vi "Drive Controller.vi"(8 "error in":errorcluster) -> ()   [LabVIEW 2018]
doc: "This VI executes continuously carrying out the current operation and responding to updates or new operation requests. It will often contain the timing or control code that is difficult to place directly in TeleOp. This VI generally opens all sensors and motors and isolates the rest of the robot code from knowing implementation details of how the operations are carried out."
uses:
  Drive Operations.ctl
  Drive Setpoints.ctl
  <vilib>/Rock Robotics/WPI/MotorControl/WPI_MotorControlOpen SPARK.vi
  <vilib>/Rock Robotics/SystemInterfaces/DIO/FPGA_DIOPWMChannel.ctl
  <vilib>/Rock Robotics/WPI/Framework/Completion Status.ctl
panel:
  in  "Interactive Values":T1
  in  "Buttons":cluster{"Execute Cmd":bool, "Abort Cmd":bool}
  out "Command Timing":cluster{"Start Time (ms)":u32, "Iterations":i32}
  out "Status":T3
  out "Current\nCmd":string
  # "Tip: The graph shows the motor setpoints. It may also be helpful to observe inputs and sensor values.\nYou may also want to display tuning or debugging controls."
  # "Interactive Command: You may fill in the settings for a command\nand schedule it with the Execute button. You can observe and abort\nany command while fine tuning the code for the controller."
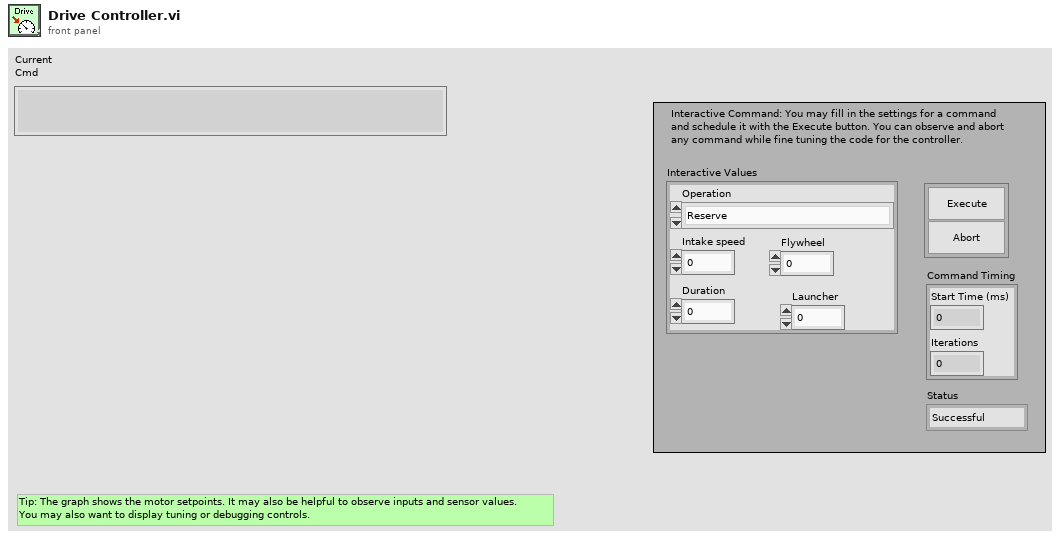
[diagram p1: front panel]
types:
  T1 = typedef "Drive Setpoints.ctl" = cluster{"Operation":T2, "Intake speed":dbl, "Duration":dbl, "Flywheel":dbl, "Launcher":dbl}
  T2 = typedef "Drive Operations.ctl" = enum16{"Reserve", "Read Current", "Immediate", "Drive for Time", "Drive for Distance"}
  T3 = typedef "Completion Status.ctl" = enum16{"Successful", "Aborted", "Incomplete"}
  T4 = typedef "FPGA_DIOPWMChannel.ctl" = enum8{"PWM 0", "PWM 1", "PWM 2", "PWM 3", "PWM 4", "PWM 5", "PWM 6", "PWM 7", "PWM 8", "PWM 9", "PWM MXP 0", "PWM MXP 1", "PWM MXP 2", "PWM MXP 3", "PWM MXP 4", "PWM MXP 5", "PWM MXP 6", "PWM MXP 7", "PWM MXP 8", "PWM MXP 9", "Invalid"}
  T5 = typedef "WPI_MotorControlDeviceRef.ctl" = cluster{"DeviceStatus":errorcluster, "Type":T6, "PWM":cluster{"PWM Channel":T4, "DeadBand":T7}, "CAN":cluster{"Device Number":u8, "SetOutput VI Ref":variant, "GetOutput VI Ref":variant, "Enable VI Ref":variant, "Disable VI Ref":variant, "Data":variant}, "Invert":bool, "DIO PWM":cluster{"PWM \"Enable\" Channel":T4, "DIOChannel":T8, "PWM Rate":dbl}}
  T6 = typedef "WPI_MotorControlType.ctl" = enum16{"PWM", "CAN", "DIO PWM"}
  T7 = typedef "WPI_PWMDeadband.ctl" = cluster{"Name":string, "maxPositivePwm":i32, "minPositivePwm":i32, "centerPwm":i32, "maxNegativePwm":i32, "minNegativePwm":i32, "angularRange":u16}
  T8 = typedef "FPGA_DIOChannel.ctl" = enum8{"DIO 0", "DIO 1", "DIO 2", "DIO 3", "DIO 4", "DIO 5", "DIO 6", "DIO 7", "DIO 8", "DIO 9", "DIO MXP 0", "DIO MXP 1", "DIO MXP 2", "DIO MXP 3", "DIO MXP 4", "DIO MXP 5", "DIO MXP 6", "DIO MXP 7", "DIO MXP 8", "DIO MXP 9", "DIO MXP 10", "DIO MXP 11", "DIO MXP 12", "DIO MXP 13", "DIO MXP 14", "DIO MXP 15", "SPI Port CS1", "SPI Port CS2", "SPI Port CS3", "SPI Port MISO", "SPI Port MOSI", "Invalid"}
  T9 = typedef "Command Status Info.ctl" = cluster{"Name":string, "Status":T3, "notifier out":T10}
  T10 = typedef "Completion Notifier.ctl" = refnum<notifier>
  T11 = cluster{"SubSystem Data":T1, cluster{"Start Time (ms)":u32, "Iterations":i32}, cluster{"Command Info":T9, "Description":string, "Default Command":T1, "queue out":refnum<queue>, "Subsystem Name":string}}
  T12 = cluster{"SubSystem Data":T1, cluster{"Start Time (ms)":u32, "Iterations":i32}, "Default Command Arguments":cluster{"Command Info":T9, "Description":string, "Default Command":T1, "queue out":refnum<queue>, "Subsystem Name":string}}
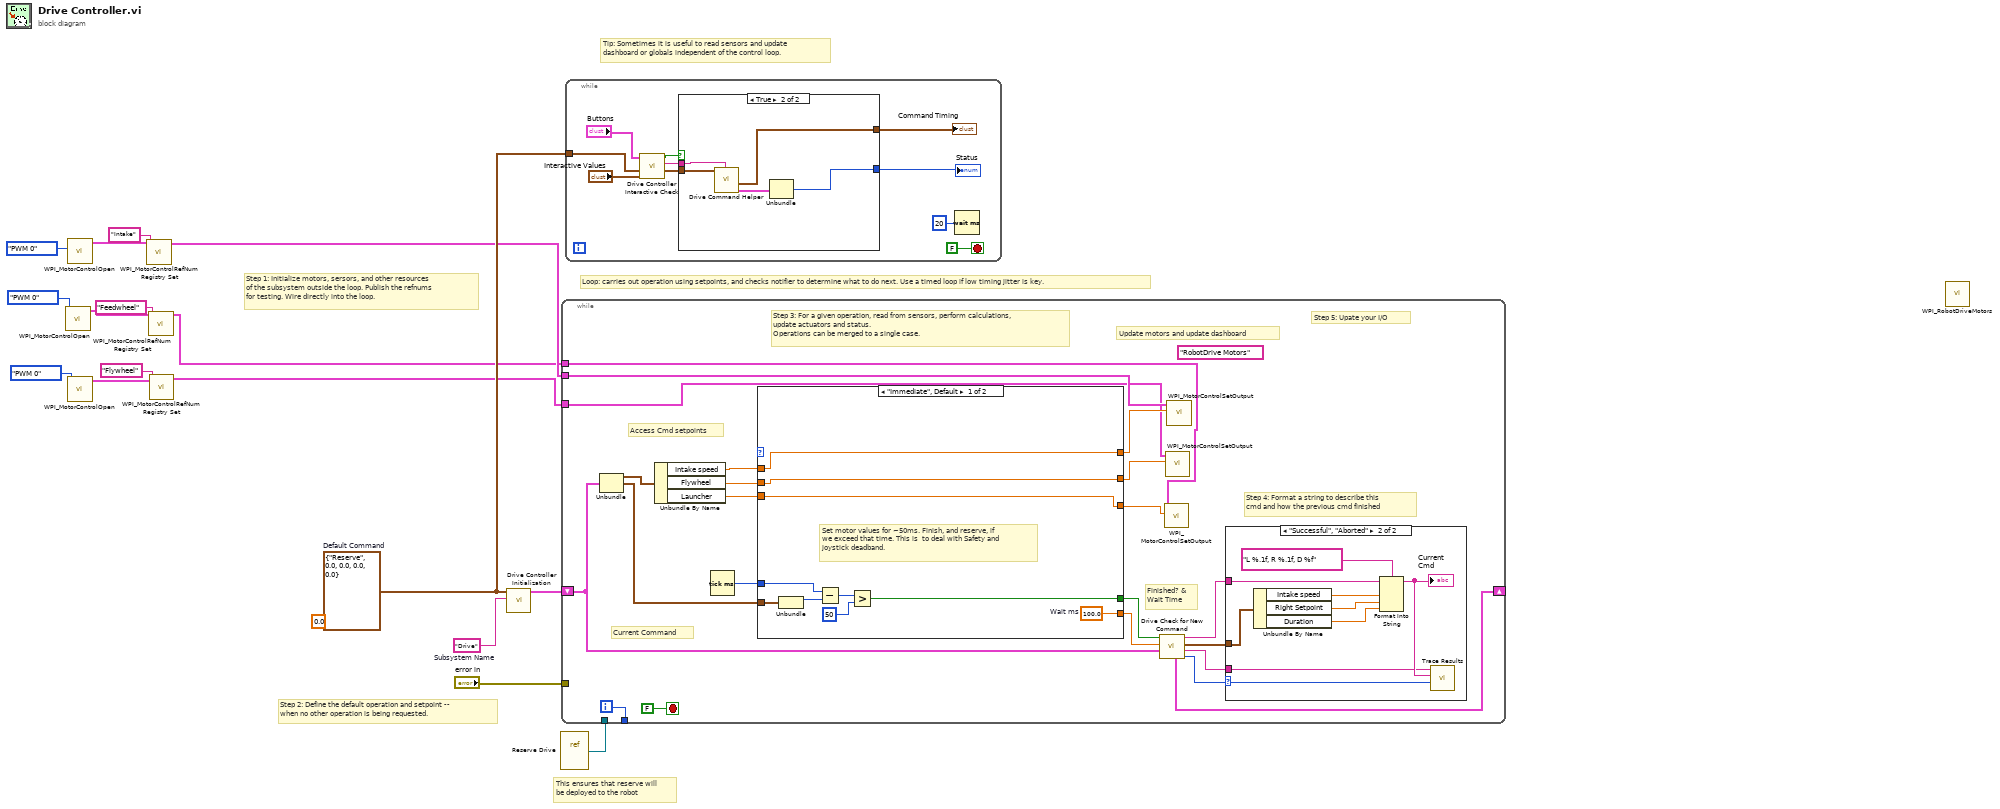
[diagram p0: block diagram]
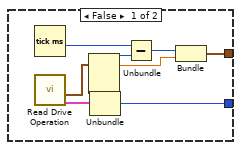
[diagram p2: hidden frame]
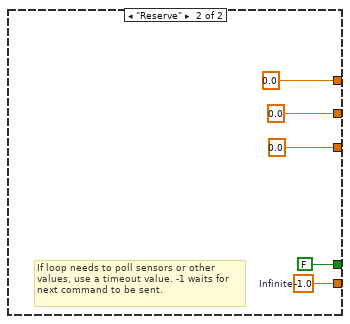
[diagram p4: hidden frame]
diagram:
  (unwired) 0.0
  w4 = T1 {"Operation"=enum."Reserve", "Intake speed"=0.0, "Duration"=0.0, "Flywheel"=0.0, "Launcher"=0.0}  # Default Command
  w8 = "Drive"  # Subsystem Name
  # "This ensures that reserve will\nbe deployed to the robot"
  # "Tip: Sometimes it is useful to read sensors and update\ndashboard or globals independent of the control loop."
  # "Step 2: Define the default operation and setpoint --\nwhen no other operation is being requested."
  # "Step 1: Initialize motors, sersors, and other resources\nof the subsystem outside the loop. Publish the refnums\nfor testing. Wire directly into the loop."
  # "Loop: carries out operation using setpoints, and checks notifier to determine what to do next. Use a timed loop if low timing jitter is key."
  n1 = call-poly <vilib>:"WPI_MotorControlOpen.vi"("PWM Channel"=FPGA_DIOPWMChannel."PWM 0") -> ("MotorControlDeviceRef"=w13:T5)  [unwired: 9 in, 1 out]
  n2 = call-poly <vilib>:"WPI_MotorControlOpen.vi"("PWM Channel"=FPGA_DIOPWMChannel."PWM 0") -> ("MotorControlDeviceRef"=w14:T5)  [unwired: 9 in, 1 out]
  n3 = call-poly <vilib>:"WPI_MotorControlOpen.vi"("PWM Channel"=FPGA_DIOPWMChannel."PWM 0") -> ("MotorControlDeviceRef"=w12:T5)  [unwired: 9 in, 1 out]
  n4 = call <vilib>:"WPI_MotorControlRefNum Registry Set.vi"("refnum name"="Intake", "MotorControlDevRef"=w14) -> ("MotorControlDevRef"=w3:T5)  [unwired: 8 in, 1 out]
  n5 = call <vilib>:"WPI_MotorControlRefNum Registry Set.vi"("refnum name"="Feedwheel", "MotorControlDevRef"=w13) -> ("MotorControlDevRef"=w2:T5)  [unwired: 8 in, 1 out]
  n6 = call <vilib>:"WPI_MotorControlRefNum Registry Set.vi"("refnum name"="Flywheel", "MotorControlDevRef"=w12) -> ("MotorControlDevRef"=w1:T5)  [unwired: 8 in, 1 out]
  n7 = call "Drive Controller Initialization.vi"("Subsystem Name"=w8, "Default Command"=w4) -> ("Current Command"=w6:T11)  [unwired: 9 in]
  n8 = vi-ref "Reserve Drive.vi"() -> (w5:refnum<vi>)
  n9 = while {
    shift-right: [w33] -> _
    shift-left: w6 -> [w26]
    tunnel: [w38] -> _
    tunnel: w3 -> [w20]
    tunnel: "error in" -> [_]
    tunnel: w5 -> [_]
    tunnel: w2 -> [w19]
    tunnel: w1 -> [w18]
    i -> [w38]
    stop <- FALSE stop-if-true
    (unwired) "RobotDrive Motors" ("Name")
    # "Step 5: Upate your I/O"
    # "Step 4: Format a string to describe this\ncmd and how the previous cmd finished"
    # "Current Command"
    # "Update motors and update dashboard"
    # "Access Cmd setpoints"
    # "Finished? &\nWait Time"
    # "Step 3: For a given operation, read from sensors, perform calculations,\nupdate actuators and status.\nOperations can be merged to a single case."
    n10 = Unbundle(w26) -> ("SubSystem Data"=w37:T1, w27:cluster{"Start Time (ms)":u32, "Iterations":i32})  [unwired: 1 out]
    n11 = Unbundle By Name(w37) -> ("Intake speed"=w36:dbl, "Flywheel"=w25:dbl, "Launcher"=w21:dbl)
    n12 = Tick Count (ms)() -> (millisecond timer value=w35:u32)
    n13 = case shown="\"Immediate\", Default" {
      selector: _ -> [_ _]
      tunnel: [w58 w63] -> w32
      tunnel: [w53 FALSE ("ignore previous (F)")] -> w31
      tunnel: w27 -> [w52 _]
      tunnel: w36 -> [w51 _]
      tunnel: w35 -> [w54 _]
      tunnel: [w51 0.0] -> w24
      tunnel: [w50 0.0] -> w23
      tunnel: [w49 0.0] -> w22
      tunnel: w25 -> [w50 _]
      tunnel: w21 -> [w49 _]
      frame "Immediate", Default {
        w58 = 100.0  # Wait ms
        # "Set motor values for ~50ms. Finish, and reserve, if\nwe exceed that time. This is  to deal with Safety and\njoystick deadband."
        n14 = Unbundle(w52) -> ("Start Time (ms)"=w55:u32)  [unwired: 1 out]
        n15 = Subtract(x=w54, y=w55) -> (x-y=w56:u32)
        n16 = Greater?(x=w56, y=u8 50 ("Left Motor")) -> (0:w53:bool)
      }
      frame "Reserve" {
        w63 = -1.0  # Infinite
        # "If loop needs to poll sensors or other\nvalues, use a timeout value. -1 waits for\nnext command to be sent."
      }
    }
    n17 = call "Drive Check for New Command.vi"("input cluster"=w26, "Wait time (ms)"=w32, "Finished?"=w31) -> ("Completion"=w34:T3, "Subsystem Name"=w28:string, "Current Command"=w29:T1, "Initial Trace String"=w30:string, "Next Command"=w33:T12)  [unwired: 4 in]
    n18 = call <vilib>:"WPI_MotorControlSetOutput.vi"("Output"=w22, "MotorControlDevRef"=w19) -> ()  [unwired: 7 in, 3 out]
    n19 = call <vilib>:"WPI_MotorControlSetOutput.vi"("Output"=w23, "MotorControlDevRef"=w18) -> ()  [unwired: 7 in, 3 out]
    n20 = call <vilib>:"WPI_MotorControlSetOutput.vi"("Output"=w24, "MotorControlDevRef"=w20) -> ()  [unwired: 7 in, 3 out]
    n21 = case shown="\"Successful\", \"Aborted\"" w34 {
      selector: w34 -> [_ w48]
      tunnel: w30 -> [_ w43]
      tunnel: w29 -> [_ w44]
      tunnel: w28 -> [_ w40]
      frame "Incomplete", Default {
        # "Continuing current command"
      }
      frame "Successful", "Aborted" {
        # "Report and setup for next command"
        n22 = Unbundle By Name(w44) -> ("Intake speed"=w46:dbl, "Right Setpoint"=w47:dbl, "Duration"=w41:dbl)
        n23 = Format Into String(format string="L %.1f, R %.1f, D %f", initial string=w43, w46, w47, w41) -> (resulting string=w42:string)  [unwired: 1 in, 1 out]
        "Current\nCmd" <- w42
        n24 = call <vilib>:"Trace Results.vi"("Status of previous command"=w48, "Description"=w42, "Subsystem"=w40) -> ()  [unwired: 9 in]
      }
    }
  }
  n25 = while {
    tunnel: w4 -> [w65]
    stop <- FALSE stop-if-true
    n26 = call "Drive Controller Interactive Check.vi"("Interactive Command In"="Interactive Values", "Default Command"=w65, "Buttons"="Buttons") -> ("Interactive Command Out"=w67:T1, "Trace String"=w68:string, "Schedule"=w69:bool)  [unwired: 6 in]
    n27 = case shown="True" w69 {
      tunnel: [w78 w86] -> w70
      tunnel: [w77 w82] -> w71
      tunnel: w68 -> [_ w84]
      tunnel: w67 -> [_ w83]
      frame False {
        n28 = Tick Count (ms)() -> (millisecond timer value=w81:u32)
        n29 = call "Read Drive Operation.vi"() -> ("Command Info"=w75:T9, "SubSystem Data"=w74:T1)  [unwired: 9 in, 1 out]
        n30 = Unbundle(w74) -> ("Operation"=w79:T2, "Intake speed"=w76:dbl)  [unwired: 3 out]
        n31 = Unbundle(w75) -> ("Status"=w78:T3)  [unwired: 2 out]
        n32 = Subtract(x=w81, y=w79) -> (x-y=w80:u32)
        n33 = Bundle(w80, "Intake speed"=w76) -> (w77:cluster{u32, "Intake speed":dbl})  [unwired: 1 in]
      }
      frame True {
        n34 = call "Drive Command Helper.vi"("Description"=w84, "SubSystem Data"=w83) -> ("Command Info Out"=w85:T9, "Command Timing"=w82:cluster{"Start Time (ms)":u32, "Iterations":i32})  [unwired: 7 in, 1 out]
        n35 = Unbundle(w85) -> ("Status"=w86:T3)  [unwired: 2 out]
      }
    }
    "Status" <- w70
    "Command Timing" <- w71
    n36 = Wait (ms)(milliseconds to wait=u32 20) -> ()  [unwired: 1 out]
  }
  n37 = call <vilib>:"WPI_RobotDriveMotors.vi"() -> ()  [unwired: 9 in, 3 out]
